vi "ex4-4.vi"() -> ()   [LabVIEW 2009]
panel:
  out "資料分布圖":cluster{dbl, dbl}(graph)
  in  "Stop":bool
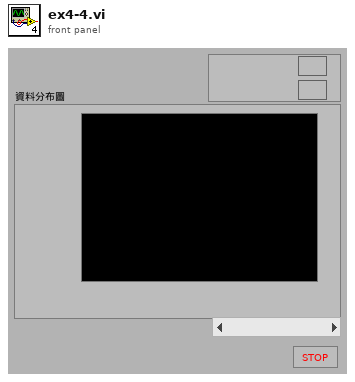
[diagram p1: front panel]
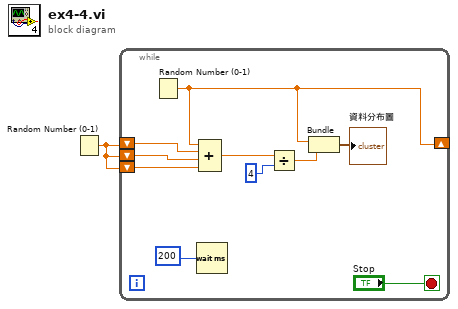
[diagram p0: block diagram]
diagram:
  n1 = Random Number (0-1)() -> (number: 0 to 1=w1:dbl)
  n2 = while {
    shift-left: w1 -> [w6]
    shift-left: w1 -> [w5]
    shift-left: w1 -> [w4]
    shift-right: [w3] -> _
    stop <- "Stop" stop-if-true
    n3 = Random Number (0-1)() -> (number: 0 to 1=w3:dbl)
    n4 = Wait (ms)(milliseconds to wait=u32 200) -> ()  [unwired: 1 out]
    n5 = Compound Arithmetic op=ADD(w3, w4, w5, w6) -> (w2:dbl)
    n6 = Divide(x=w2, y=4) -> (x/y=w9:dbl)
    n7 = Bundle(w3, w9) -> (→"資料分布圖":cluster{dbl, dbl})  [unwired: 1 in]
  }
